vi "name.get.vi"(11 "test-device in":refnum<class "test-device.lvclass">) -> (2 "name":string, 3 "test-device out":refnum<class "test-device.lvclass">)   [LabVIEW 2020, in "test-device.lvclass"]
uses:
  test-device.lvclass
  test-device.lvclass/test-device.ctl
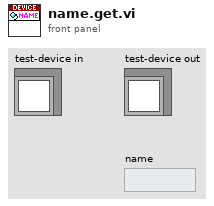
[diagram p1: front panel]
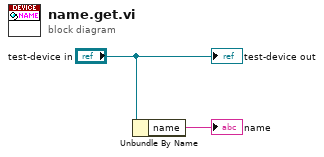
[diagram p0: block diagram]
diagram:
  n1 = Unbundle By Name("test-device in") -> ("name"=→"name":string)
  "test-device out" <- "test-device in"
